vi "Agilent SNA Convert Form 3 Data.vi"(6 "Measurement Format (Log Mag)":T1, 8 "Raw Data Point":string) -> (0 "Number":cdb)   [LabVIEW 2011]
uses:
  SNA Measurement Format.ctl
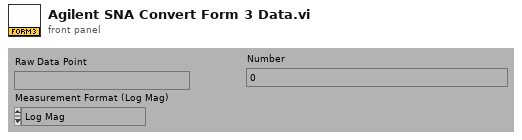
[diagram p1: front panel]
types:
  T1 = typedef "SNA Measurement Format.ctl" = enum32{"Log Mag", "Normalized Log Mag", "SWR", "Linear Mag", "Power Out"}
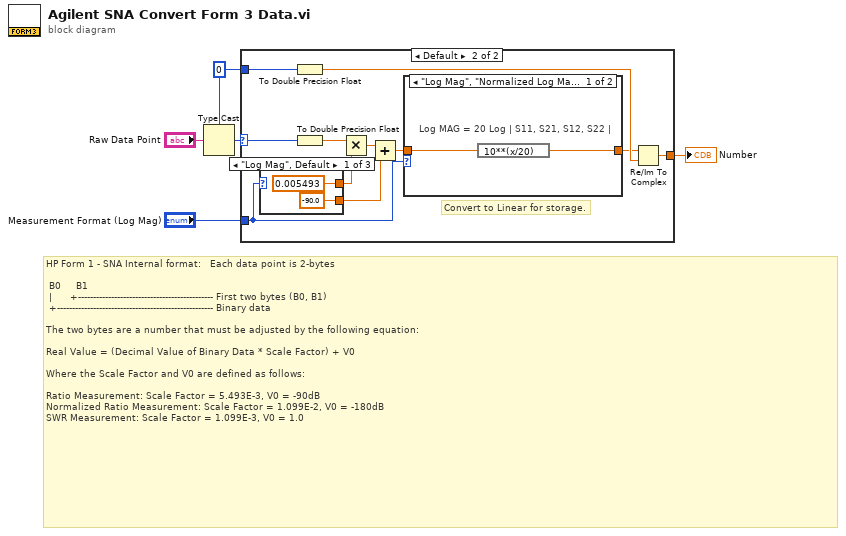
[diagram p0: block diagram]
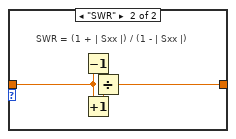
[diagram p3: hidden frame]
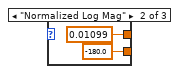
[diagram p4: hidden frame]
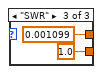
[diagram p5: hidden frame]
diagram:
  w1 = i16 0
  # "HP Form 1 - SNA Internal format:   Each data point is 2-bytes\n\n B0     B1\n |      +--------------------------------------------- First two bytes (B0, B1)\n +---------------------------------------------------- Binary data\n\nThe two bytes are a number that must be adjusted by the following equation:\n\nReal Value = (Decimal Value of Binary Data * Scale Factor) + V0\n\nWhere the Scale Factor and V0 are defined as follows:\n\nRatio Measurement: Scale Factor = 5.493E-3, V0 = -90dB\nNormalized Ratio Measurement: Scale Factor = 1.099E-2, V0 = -180dB\nSWR Measurement: Scale Factor = 1.099E-3, V0 = 1.0"
  n1 = Type Cast(type=w1, x="Raw Data Point") -> (*(type *) &x=w2:i16)
  n2 = case shown="Default" w2 {
    selector: w2 -> [_ w7]
    tunnel: [_ w15] -> w5
    tunnel: "Measurement Format (Log Mag)" -> [_ w8]
    tunnel: w1 -> [_ w6]
    frame 0 {
    }
    frame Default {
      # "Convert to Linear for storage."
      n3 = case shown="\"Log Mag\", Default" w8 {
        tunnel: [0.005493 0.01099 0.001099] -> w13
        tunnel: [-90.0 -180.0 1.0] -> w12
        frame "Log Mag", Default {
        }
        frame "Normalized Log Mag" {
        }
        frame "SWR" {
        }
      }
      n4 = To Double Precision Float(number=w6) -> (double precision float=w16:dbl)
      n5 = To Double Precision Float(number=w7) -> (double precision float=w14:dbl)
      n6 = Multiply(x=w14, y=w13) -> (x*y=w11:dbl)
      n7 = Add(x=w11, y=w12) -> (x+y=w9:dbl)
      n8 = case shown="\"Log Mag\", \"Normalized Log Mag\", Default" w8 {
        tunnel: w9 -> [w18 w20]
        tunnel: [w17 w19] -> w10
        frame "Log Mag", "Normalized Log Mag", Default {
          # "Log MAG = 20 Log | S11, S21, S12, S22 |"
          n9 = expression code="10**(x/20)"(w18) -> (w17:dbl)
        }
        frame "SWR" {
          # "SWR = (1 + | Sxx |) / (1 - | Sxx |)"
          n10 = Decrement(x=w20) -> (x-1=w21:dbl)
          n11 = Increment(x=w20) -> (x+1=w22:dbl)
          n12 = Divide(x=w21, y=w22) -> (x/y=w19:dbl)
        }
      }
      n13 = Re/Im To Complex(1:w16, 2:w10) -> (0:w15:cdb)
    }
  }
  "Number" <- w5
